vi "Disable All Controls.vi"(8 "error in (no error)":errorcluster, 10 "Disabled":T1(ring), 11 "Simulated Sensor Interface Actor in":refnum<class "Simulated Sensor Interface Actor.lvclass">) -> (0 "error out":errorcluster, 3 "Simulated Sensor Interface Actor out":refnum<class "Simulated Sensor Interface Actor.lvclass">)   [LabVIEW 2019, in "Simulated Sensor Interface Actor.lvlib" / "Simulated Sensor Interface Actor.lvclass"]
uses:
  Simulated Sensor Interface Actor.lvclass
  Simulated Sensor Interface Actor.lvclass/Simulated Sensor Interface Actor.ctl
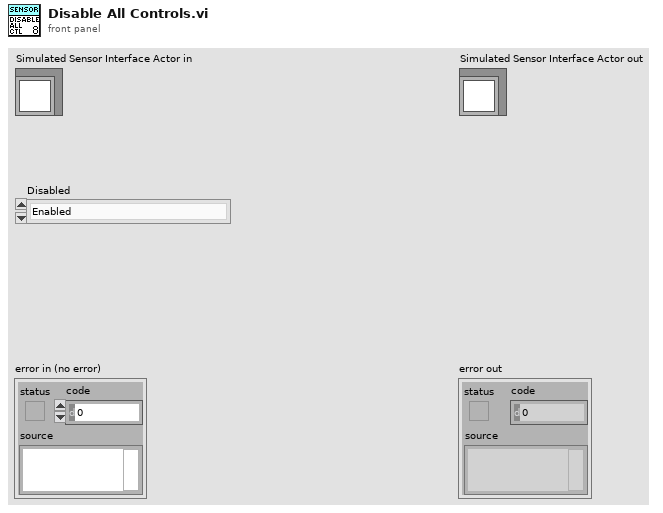
[diagram p1: front panel]
types:
  T1 = enum8{"Enabled", "Disabled", "Disabled and Grayed Out"}
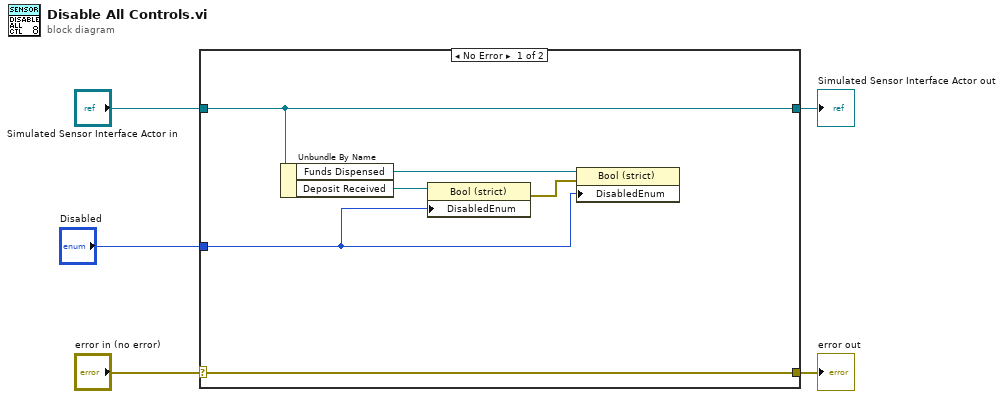
[diagram p0: block diagram]
diagram:
  n1 = case shown="No Error" "error in (no error)" {
    selector: "error in (no error)" -> [w11 w13]
    tunnel: [w11 w13] -> w4
    tunnel: [w10 w12] -> w2
    tunnel: "Simulated Sensor Interface Actor in" -> [w10 w12]
    tunnel: "Disabled" -> [w6 _]
    frame No Error {
      n2 = Unbundle By Name(w10) -> ("Funds Dispensed"=w7:refnum<vi>, "Deposit Received"=w9:refnum<vi>)
      n3 = property class="Bool (strict)"(reference=w9, "DisabledEnum"=w6) -> (error out=w8:errorcluster)  [unwired: 1 in, 1 out]
      n4 = property class="Bool (strict)"(reference=w7, error in=w8, "DisabledEnum"=w6) -> ()  [unwired: 2 out]
    }
    frame Error {
    }
  }
  "error out" <- w4
  "Simulated Sensor Interface Actor out" <- w2
